vi "close visa.vi"(8 "error in (no error)":errorcluster, 11 "Cypress in":refnum<class "Cypress.lvclass">) -> (0 "error out":errorcluster, 3 "Cypress out":refnum<class "Cypress.lvclass">)   [LabVIEW 2020, in "Cypress.lvclass"]
doc: "Override del papa close visa"
uses:
  Cypress.lvclass
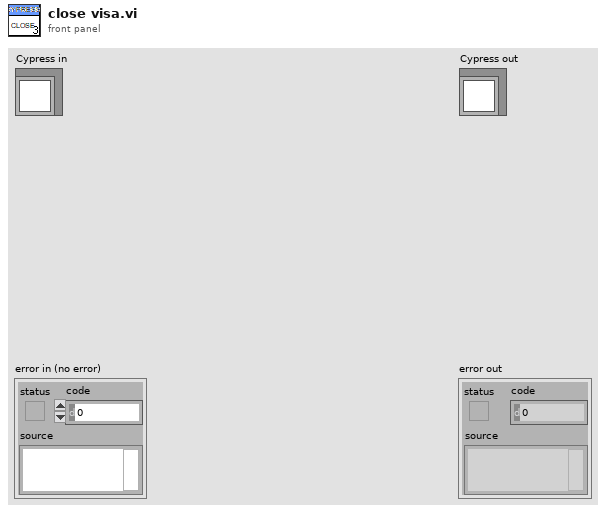
[diagram p1: front panel]
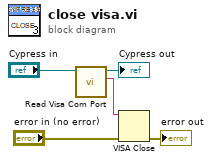
[diagram p0: block diagram]
diagram:
  n1 = call-dynamic "Read Visa Com Port.vi"("Serial Device in"="Cypress in") -> ("Visa Com Port"=w3:string, "Serial Device out"=→"Cypress out":refnum<class "Cypress.lvclass">)  [unwired: 8 in, 1 out]
  n2 = VISA Close(VISA resource name=w3, error in (no error)="error in (no error)") -> (error out=→"error out":errorcluster)
